vi "Change Setting.vi"(7 "Data":string, 8 "error in (no error)":errorcluster, 9 "Device and Axis":string, 10 "Setting":string, 11 "VISA resource name":refnum<visa-resource-name>) -> (0 "error out":errorcluster, 3 "VISA resource name out":refnum<visa-resource-name>)   [LabVIEW 2018, in "Zaber A Series.lvlib"]
doc: "Changes a setting from the device. Omitting the Device and Axis will change the settings of all connected devices. See a list of settings available here: http://www.zaber.com/wiki/Manuals/ASCII_Protocol_Manual#Device_Settings. You do not need to include the 'set' command with this VI, you only need to input the setting you'd like to change. \n\nThe Detect Devices VI is designed to provide an easy list of valid Device and Axis inputs. \n\nThis VI requires that the Initialize VI has been called with the same serial port."
uses:
  Zaber A Series.lvlib
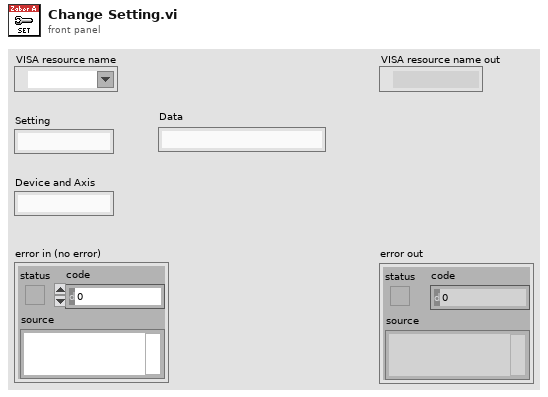
[diagram p1: front panel]
types:
  T1 = cluster{"Device":string, "Axis":string, "Reply Flag":string, "Status":string, "Warning Flags":string, "Data":string}[]
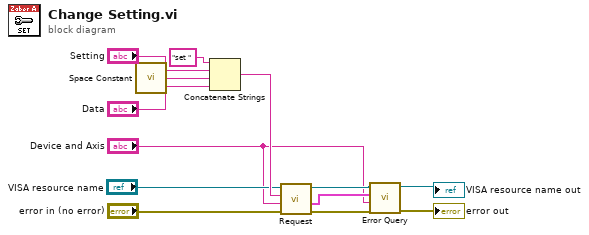
[diagram p0: block diagram]
diagram:
  n1 = call <vilib>:"Space Constant.vi"() -> ("String"=w11:string)
  n2 = Concatenate Strings("set " ("string"), "Setting", w11, "Data") -> (w9:string)
  n3 = call "Request.vi"("error in (no error)"="error in (no error)", "Device and Axis"="Device and Axis", "Command String"=w9, "VISA resource name"="VISA resource name") -> ("error out"=w4:errorcluster, "Response Bundle Array"=w2:T1, "VISA resource name out"=w6:refnum<visa-resource-name>)  [unwired: 2 in, 3 out]
  n4 = call "Error Query.vi"("error in (no error)"=w4, "Device and Axis"="Device and Axis", "Previous Response Bundle Array"=w2, "VISA resource name"=w6) -> ("error out"=→"error out":errorcluster, "VISA resource name out"=→"VISA resource name out":refnum<visa-resource-name>)  [unwired: 4 in, 2 out]
